vi "Rx Init.vi"(8 "error in (no error)":errorcluster, 9 "Channel Number":u32, 10 "signal list":refnum<k21>[](array[refnum])=["CANEventSignal1\nNIXNET_example.CAN_Cluster", "CANCyclicSignal2\nnixnet_example.CAN_Cluster"], 11 "FPGA Refnum":T1) -> (0 "error out":errorcluster, 3 "Rx Session":T2)   [LabVIEW 2020, in "985x Support Addon Engine.lvlib"]
uses:
  985x Support Addon Engine.lvlib
  Types/Rx Session.ctl
  Types/FPGA Refnum.ctl
  <vilib>/xnet/xnet.llb/XNET Create Session (Conversion).vi
  <resource>/objmgr/xnet.rc
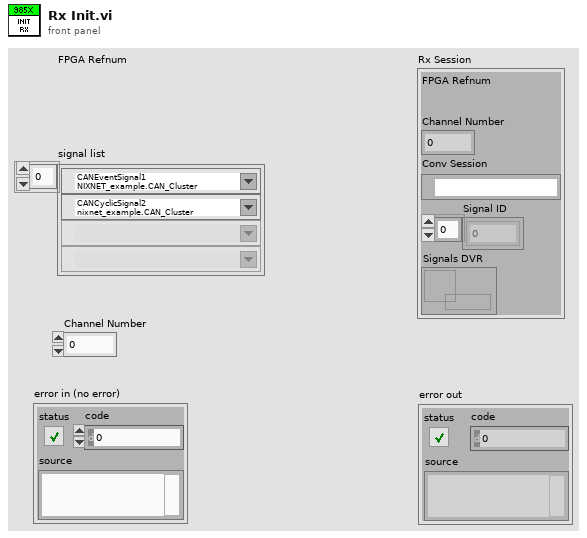
[diagram p1: front panel]
types:
  T1 = typedef "985x Support Addon Engine.lvlib/FPGA Refnum.ctl" = refnum<k20>
  T2 = typedef "985x Support Addon Engine.lvlib/Rx Session.ctl" = cluster{"FPGA Refnum":T1, "Channel Number":u32, "Conv Session":refnum<k21>, "Signal ID":u32[], "Signals DVR":refnum<data-value>}
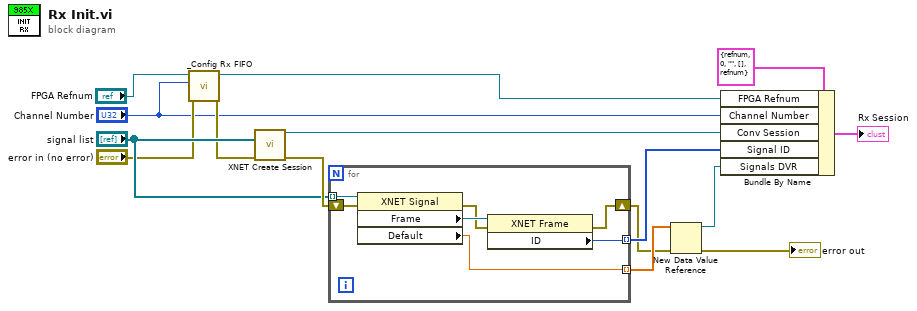
[diagram p0: block diagram]
diagram:
  n1 = call "_Config Rx FIFO.vi"("error in (no error)"="error in (no error)", "Channel Number"="Channel Number", "Refnum in"="FPGA Refnum") -> ("error out"=w2:errorcluster, "Refnum out"=w3:T1)  [unwired: 7 in]
  n2 = call-poly <vilib>:"XNET Create Session.vi"("signal list"="signal list", "error in (no error)"=w2) -> ("session out"=w13:refnum<k21>, "error out"=w15:errorcluster)  [unwired: 12 out]
  n3 = for {
    tunnel: "signal list" -> [w22] mode=indexing
    shift-right: [w20] -> w8
    shift-left: w15 -> [w21]
    tunnel: [w17] -> w11 mode=indexing
    tunnel: [w16] -> w9 mode=indexing
    n4 = property class="XNET Signal"(reference=w22, error in=w21) -> (error out=w18:errorcluster, "Frame"=w19:refnum<k21>, "Default"=w16:dbl)  [unwired: 1 out]
    n5 = property class="XNET Frame"(reference=w19, error in=w18) -> (error out=w20:errorcluster, "ID"=w17:u32)  [unwired: 1 out]
  }
  n6 = New Data Value Reference(data value=w9, error in=w8) -> (data value reference=w6:refnum<data-value>, error out=→"error out":errorcluster)
  n7 = Bundle By Name(cluster=T2 {"FPGA Refnum"=refnum, "Channel Number"=0, "Conv Session"="", "Signal ID"=[], "Signals DVR"=refnum} ("Rx Session"), "FPGA Refnum"=w3, "Channel Number"="Channel Number", "Conv Session"=w13, "Signal ID"=w11, "Signals DVR"=w6) -> (→"Rx Session":T2)
